vi "Run.vi"(8 "error in (no error)":errorcluster, 11 "SPARC4_GUI in":refnum<class "SPARC4_GUI.lvclass">) -> (0 "error out":errorcluster, 3 "SPARC4_GUI out":refnum<class "SPARC4_GUI.lvclass">)   [LabVIEW 2018, in "SPARC4_GUI.lvclass"]
uses:
  SPARC4_GUI.lvclass
  SPARC4_GUI.lvclass/SPARC4_GUI.ctl
  State Machine/State Machine.lvclass
  Stream/Stream.lvclass
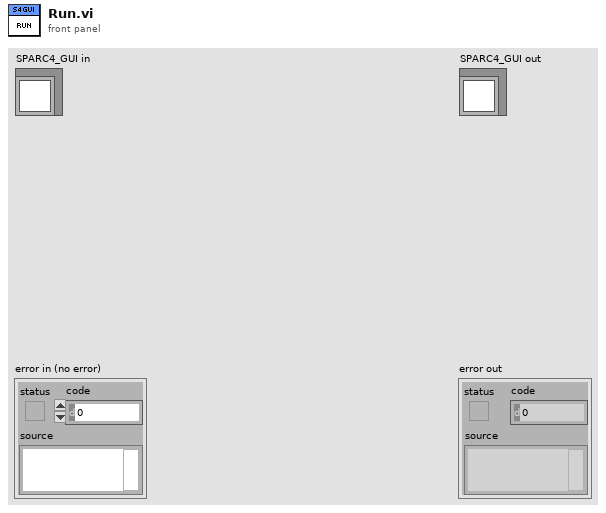
[diagram p1: front panel]
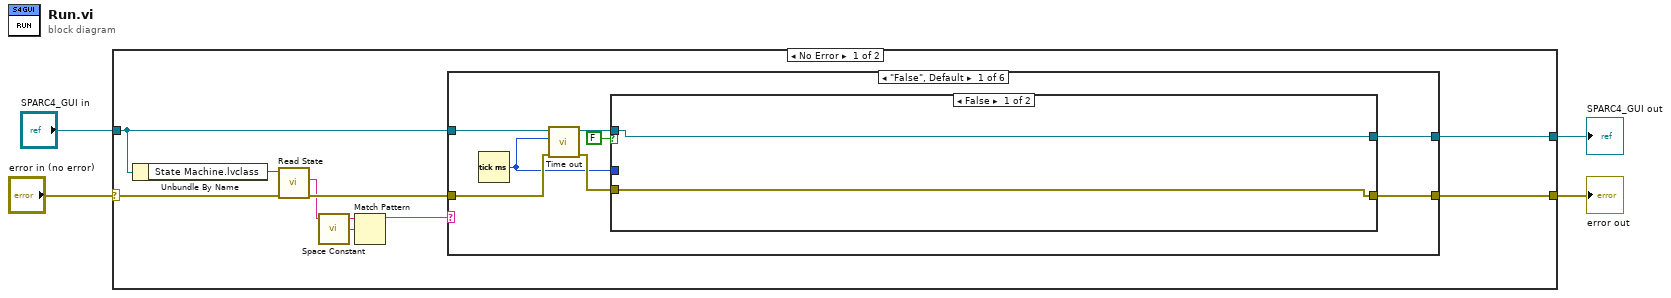
[diagram p0: block diagram]
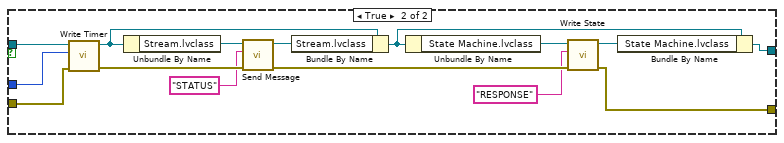
[diagram p2: hidden frame]
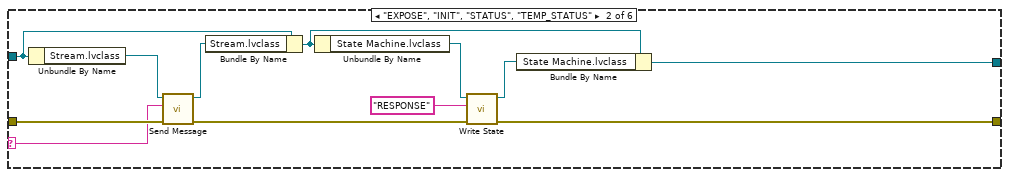
[diagram p3: hidden frame]
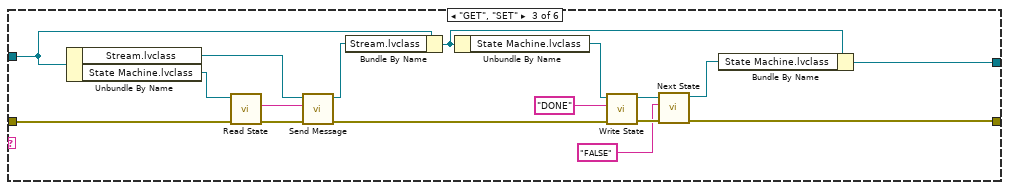
[diagram p4: hidden frame]
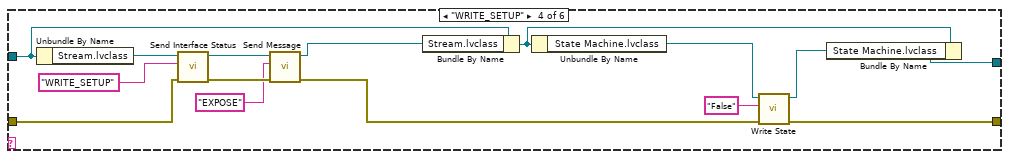
[diagram p5: hidden frame]
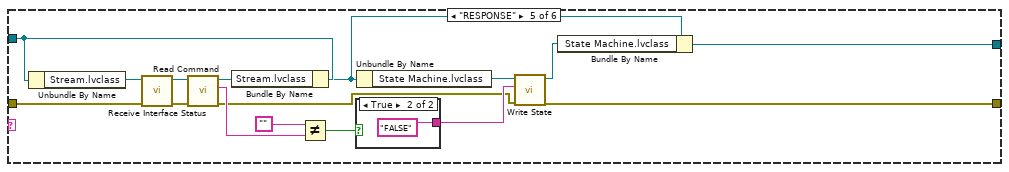
[diagram p6: hidden frame]
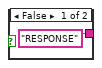
[diagram p7: hidden frame]
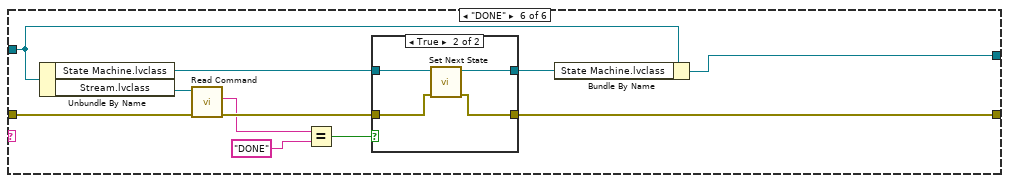
[diagram p8: hidden frame]
diagram:
  n1 = case shown="No Error" "error in (no error)" {
    selector: "error in (no error)" -> [w11 w119]
    tunnel: [w13 w119] -> w3
    tunnel: [w8 w118] -> w1
    tunnel: "SPARC4_GUI in" -> [w9 w118]
    frame No Error {
      n2 = Unbundle By Name(w9) -> ("State Machine.lvclass"=w12:refnum<class "State Machine.lvclass">)
      n3 = call-dynamic "Read State.vi"("error in (no error)"=w11, "State Machine in"=w12) -> ("error out"=w10:errorcluster, "State"=w6:string)  [unwired: 7 in, 1 out]
      n4 = call <vilib>:"Space Constant.vi"() -> ("String"=w7:string)
      n5 = Match Pattern(string=w6, regular expression=w7) -> (before substring=w5:string)  [unwired: 1 in, 3 out]
      n6 = case shown="\"False\", Default" w5 {
        selector: w5 -> [_ w39 _ _ _ _]
        tunnel: w10 -> [w20 w49 w52 w74 w91 w110]
        tunnel: [w16 w42 w56 w78 w97 w102] -> w13
        tunnel: w9 -> [w21 w48 w61 w80 w98 w104]
        tunnel: [w15 w45 w62 w79 w94 w101] -> w8
        frame "False", Default {
          n7 = Tick Count (ms)() -> (millisecond timer value=w17:u32)
          n8 = call "Time out"("error in (no error)"=w20, "New Time"=w17, "SPARC4_GUI in"=w21) -> ("error out"=w18:errorcluster, "SPARC4_GUI out"=w19:refnum<class "SPARC4_GUI.lvclass">)  [unwired: 6 in, 1 out]
          n9 = case shown="False" FALSE {
            tunnel: w19 -> [w23 w38]
            tunnel: w18 -> [w22 w37]
            tunnel: w17 -> [_ w36]
            tunnel: [w22 w26] -> w16
            tunnel: [w23 w25] -> w15
            frame False {
            }
            frame True {
              n10 = call "Write Timer.vi"("error in (no error)"=w37, "Timer"=w36, "SPARC4_GUI in"=w38) -> ("error out"=w32:errorcluster, "SPARC4_GUI out"=w33:refnum<class "SPARC4_GUI.lvclass">)  [unwired: 7 in]
              n11 = Unbundle By Name(w33) -> ("Stream.lvclass"=w34:refnum<class "Stream.lvclass">)
              n12 = call "Send Message.vi"("error in (no error)"=w32, "Message"="STATUS" ("New_State"), "Stream in"=w34) -> ("error out"=w29:errorcluster, "Stream out"=w35:refnum<class "Stream.lvclass">)  [unwired: 7 in]
              n13 = Bundle By Name(cluster=w33, "Stream.lvclass"=w35) -> (w27:refnum<class "SPARC4_GUI.lvclass">)
              n14 = Unbundle By Name(w27) -> ("State Machine.lvclass"=w30:refnum<class "State Machine.lvclass">)
              n15 = call-dynamic "Write State.vi"("error in (no error)"=w29, "State"="RESPONSE" ("New_State"), "State Machine in"=w30) -> ("error out"=w26:errorcluster, "State Machine out"=w28:refnum<class "State Machine.lvclass">)  [unwired: 7 in]
              n16 = Bundle By Name(cluster=w27, "State Machine.lvclass"=w28) -> (w25:refnum<class "SPARC4_GUI.lvclass">)
            }
          }
        }
        frame "EXPOSE", "INIT", "STATUS", "TEMP_STATUS" {
          n17 = Unbundle By Name(w48) -> ("Stream.lvclass"=w50:refnum<class "Stream.lvclass">)
          n18 = call "Send Message.vi"("error in (no error)"=w49, "Message"=w39, "Stream in"=w50) -> ("error out"=w41:errorcluster, "Stream out"=w47:refnum<class "Stream.lvclass">)  [unwired: 7 in]
          n19 = Bundle By Name(cluster=w48, "Stream.lvclass"=w47) -> (w46:refnum<class "SPARC4_GUI.lvclass">)
          n20 = Unbundle By Name(w46) -> ("State Machine.lvclass"=w44:refnum<class "State Machine.lvclass">)
          n21 = call-dynamic "Write State.vi"("error in (no error)"=w41, "State"="RESPONSE" ("New_State"), "State Machine in"=w44) -> ("error out"=w42:errorcluster, "State Machine out"=w43:refnum<class "State Machine.lvclass">)  [unwired: 7 in]
          n22 = Bundle By Name(cluster=w46, "State Machine.lvclass"=w43) -> (w45:refnum<class "SPARC4_GUI.lvclass">)
        }
        frame "GET", "SET" {
          n23 = Unbundle By Name(w61) -> ("Stream.lvclass"=w64:refnum<class "Stream.lvclass">, "State Machine.lvclass"=w54:refnum<class "State Machine.lvclass">)
          n24 = call-dynamic "Read State.vi"("error in (no error)"=w52, "State Machine in"=w54) -> ("error out"=w53:errorcluster, "State"=w51:string)  [unwired: 7 in, 1 out]
          n25 = call "Send Message.vi"("error in (no error)"=w53, "Message"=w51, "Stream in"=w64) -> ("error out"=w67:errorcluster, "Stream out"=w65:refnum<class "Stream.lvclass">)  [unwired: 7 in]
          n26 = Bundle By Name(cluster=w61, "Stream.lvclass"=w65) -> (w66:refnum<class "SPARC4_GUI.lvclass">)
          n27 = Unbundle By Name(w66) -> ("State Machine.lvclass"=w60:refnum<class "State Machine.lvclass">)
          n28 = call-dynamic "Write State.vi"("error in (no error)"=w67, "State"="DONE" ("New_State"), "State Machine in"=w60) -> ("error out"=w59:errorcluster, "State Machine out"=w58:refnum<class "State Machine.lvclass">)  [unwired: 7 in]
          n29 = call "Next State.vi"("error in (no error)"=w59, "New_State"="FALSE", "State Machine in"=w58) -> ("error out"=w56:errorcluster, "State Machine out"=w57:refnum<class "State Machine.lvclass">)  [unwired: 7 in]
          n30 = Bundle By Name(cluster=w66, "State Machine.lvclass"=w57) -> (w62:refnum<class "SPARC4_GUI.lvclass">)
        }
        frame "WRITE_SETUP" {
          n31 = Unbundle By Name(w80) -> ("Stream.lvclass"=w75:refnum<class "Stream.lvclass">)
          n32 = call "Send Interface Status.vi"("error in (no error)"=w74, "Message"="WRITE_SETUP" ("New_State"), "Stream in"=w75) -> ("error out"=w69:errorcluster, "Stream out"=w72:refnum<class "Stream.lvclass">)  [unwired: 7 in]
          n33 = call "Send Message.vi"("error in (no error)"=w69, "Message"="EXPOSE" ("New_State"), "Stream in"=w72) -> ("error out"=w70:errorcluster, "Stream out"=w71:refnum<class "Stream.lvclass">)  [unwired: 7 in]
          n34 = Bundle By Name(cluster=w80, "Stream.lvclass"=w71) -> (w81:refnum<class "SPARC4_GUI.lvclass">)
          n35 = Unbundle By Name(w81) -> ("State Machine.lvclass"=w82:refnum<class "State Machine.lvclass">)
          n36 = call-dynamic "Write State.vi"("error in (no error)"=w70, "State"="False" ("New_State"), "State Machine in"=w82) -> ("error out"=w78:errorcluster, "State Machine out"=w77:refnum<class "State Machine.lvclass">)  [unwired: 7 in]
          n37 = Bundle By Name(cluster=w81, "State Machine.lvclass"=w77) -> (w79:refnum<class "SPARC4_GUI.lvclass">)
        }
        frame "RESPONSE" {
          n38 = Unbundle By Name(w98) -> ("Stream.lvclass"=w92:refnum<class "Stream.lvclass">)
          n39 = call "Receive Interface Status.vi"("error in (no error)"=w91, "Stream in"=w92) -> ("error out"=w90:errorcluster, "Stream out"=w89:refnum<class "Stream.lvclass">)  [unwired: 8 in]
          n40 = call "Read Command.vi"("error in (no error)"=w90, "Stream in"=w89) -> ("error out"=w83:errorcluster, "Command"=w88:string, "Stream out"=w85:refnum<class "Stream.lvclass">)  [unwired: 7 in]
          n41 = Bundle By Name(cluster=w98, "Stream.lvclass"=w85) -> (w95:refnum<class "SPARC4_GUI.lvclass">)
          n42 = Not Equal?(x="", y=w88) -> (x != y?=w86:bool)
          n43 = case shown="True" w86 {
            tunnel: ["RESPONSE" "FALSE"] -> w84
            frame False {
            }
            frame True {
            }
          }
          n44 = Unbundle By Name(w95) -> ("State Machine.lvclass"=w96:refnum<class "State Machine.lvclass">)
          n45 = call-dynamic "Write State.vi"("error in (no error)"=w83, "State"=w84, "State Machine in"=w96) -> ("error out"=w97:errorcluster, "State Machine out"=w93:refnum<class "State Machine.lvclass">)  [unwired: 7 in]
          n46 = Bundle By Name(cluster=w95, "State Machine.lvclass"=w93) -> (w94:refnum<class "SPARC4_GUI.lvclass">)
        }
        frame "DONE" {
          n47 = Unbundle By Name(w104) -> ("State Machine.lvclass"=w105:refnum<class "State Machine.lvclass">, "Stream.lvclass"=w111:refnum<class "Stream.lvclass">)
          n48 = call "Read Command.vi"("error in (no error)"=w110, "Stream in"=w111) -> ("error out"=w109:errorcluster, "Command"=w106:string)  [unwired: 7 in, 1 out]
          n49 = Equal?(x=w106, y="DONE") -> (x = y?=w108:bool)
          n50 = case shown="True" w108 {
            tunnel: [w113 w114] -> w102
            tunnel: w109 -> [w113 w115]
            tunnel: w105 -> [w112 w117]
            tunnel: [w112 w116] -> w103
            frame False {
            }
            frame True {
              n51 = call "Set Next State.vi"("error in (no error)"=w115, "State Machine in"=w117) -> ("error out"=w114:errorcluster, "State Machine out"=w116:refnum<class "State Machine.lvclass">)  [unwired: 8 in]
            }
          }
          n52 = Bundle By Name(cluster=w104, "State Machine.lvclass"=w103) -> (w101:refnum<class "SPARC4_GUI.lvclass">)
        }
      }
    }
    frame Error {
    }
  }
  "error out" <- w3
  "SPARC4_GUI out" <- w1
